vi "NewShooterStateController.vi"(1 "Selected State (In)":string) -> (0 "Selected State (Out)":string)   [LabVIEW 2019]
uses:
  dsinstructions.vi
  outputs.vi
  sensors.vi
  constants.vi
  dsdata.vi
panel:
  in  "Settling Time (ms)":u32=500
  in  "Max Acceptable Robot Speed (ft/s)":dbl=5.0
  in  "Acceptable Shooter Error Fraction":dbl=0.1
  in  "Shooter Prespin (ms)":u32=7000
  in  "Shooter Off Delay (ms)":u32=1000
  in  "Max Range (in)":dbl=1000.0
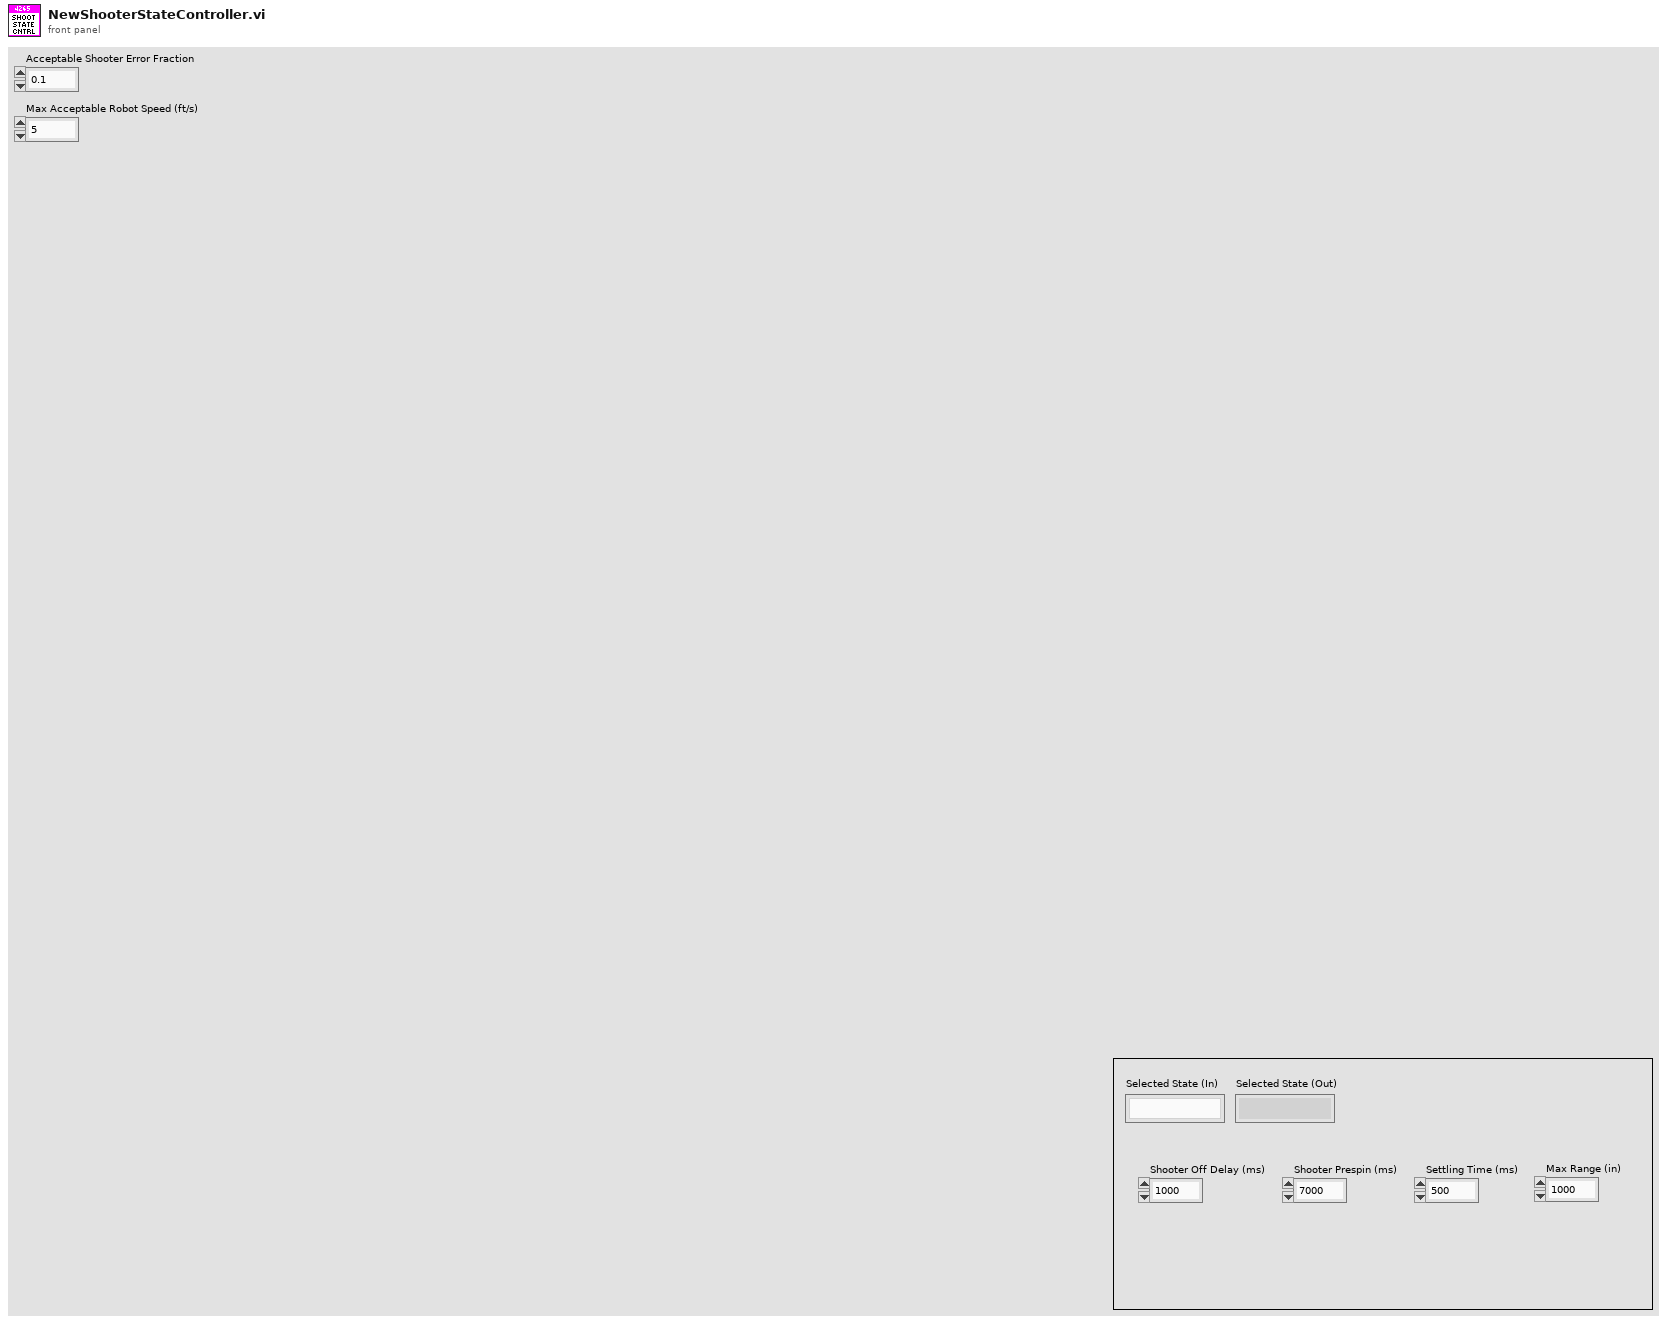
[diagram p1: front panel]
types:
  T1 = enum16{"Center", "North", "NorthWest", "West", "SouthWest", "South", "SouthEast", "East", "NorthEast"}
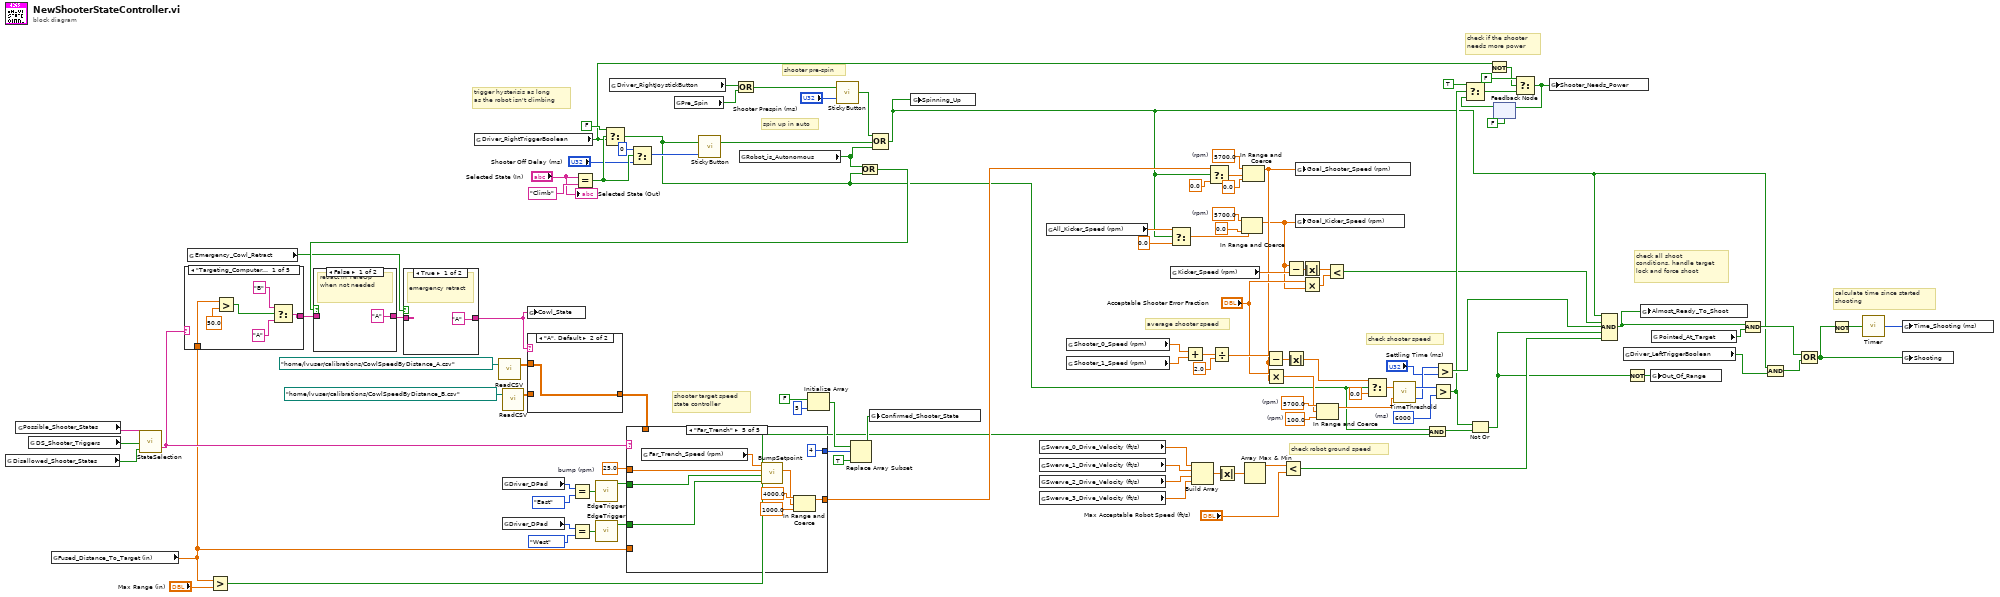
[diagram p0: block diagram]
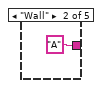
[diagram p4: hidden frame]
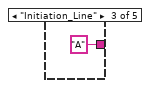
[diagram p5: hidden frame]
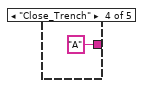
[diagram p6: hidden frame]
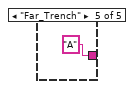
[diagram p7: hidden frame]
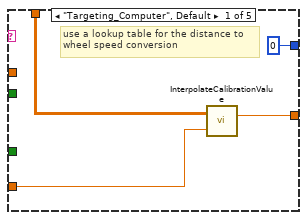
[diagram p9: hidden frame]
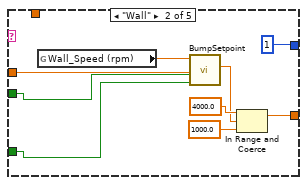
[diagram p10: hidden frame]
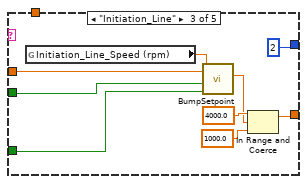
[diagram p11: hidden frame]
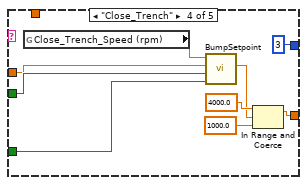
[diagram p12: hidden frame]
diagram:
  w33 = 100.0  # (rpm)
  w34 = 5700.0  # (rpm)
  w42 = 5700.0  # (rpm)
  w5 = 5700.0  # (rpm)
  w45 = u32 6000  # (ms)
  w96 = 25.0  # bump (rpm)
  # "calculate time since started\nshooting"
  # "check all shoot\nconditions, handle target\nlock and force shoot"
  # "average shooter speed"
  # "check shooter speed"
  # "check robot ground speed"
  # "check if the shooter\nneeds more power"
  # "shooter pre-spin"
  # "spin up in auto"
  # "trigger hysterisis as long\nas the robot isn't climbing"
  # "shooter target speed\nstate controller"
  n1 = global read "outputs.vi" "Disallowed_Shooter_States"() -> (w95:bool[])
  n2 = global read "constants.vi" "Possible_Shooter_States"() -> (w113:string[])
  n3 = global read "dsinstructions.vi" "DS_Shooter_Triggers"() -> (w112:bool[])
  n4 = global read "sensors.vi" "Fused_Distance_To_Target (in)"() -> (w86:dbl)
  n5 = call "StateSelection.vi"("Disallowed States"=w95, "State Triggers"=w112, "State Names"=w113) -> ("Selected State"=w87:string)
  n6 = case shown="\"Targeting_Computer\", Default" w87 {
    tunnel: [w114 "A" ("A,B,C") "A" ("A,B,C") "A" ("A,B,C") "A" ("A,B,C")] -> w89
    tunnel: w86 -> [w115 _ _ _ _]
    frame "Targeting_Computer", Default {
      n7 = Greater?(x=w115, y=50.0) -> (0:w119:bool)
      n8 = Select(t="B", s=w119, f="A") -> (s? t:f=w114:string)
    }
    frame "Wall" {
    }
    frame "Initiation_Line" {
    }
    frame "Close_Trench" {
    }
    frame "Far_Trench" {
    }
  }
  n9 = global read "dsdata.vi" "Emergency_Cowl_Retract"() -> (w70:bool)
  n10 = Greater?(x=w86, y="Max Range (in)") -> (0:w20:bool)
  n11 = global read "dsinstructions.vi" "Driver_RightTriggerBoolean"() -> (w63:bool)
  n12 = call "ReadCSV.vi"("File Path (.csv)"=path "/home/lvuser/calibrations/CowlSpeedByDistance_A.csv" ("path")) -> ("Data (index by row)"=w92:dbl[][])  [unwired: 1 in, 1 out]
  n13 = call "ReadCSV.vi"("File Path (.csv)"=path "/home/lvuser/calibrations/CowlSpeedByDistance_B.csv" ("path")) -> ("Data (index by row)"=w91:dbl[][])  [unwired: 1 in, 1 out]
  n14 = global read "dsinstructions.vi" "Driver_DPad"() -> (w104:T1)
  n15 = global read "dsinstructions.vi" "Driver_DPad"() -> (w100:T1)
  n16 = Equal?(x=w104, y=T1."East" ("Driver_DPad")) -> (x = y?=w102:bool)
  n17 = Equal?(x=w100, y=T1."West" ("Driver_DPad")) -> (x = y?=w99:bool)
  n18 = Equal?(x="Selected State (In)", y="Climb") -> (x = y?=w83:bool)
  n19 = call "EdgeTrigger.vi"("Input Signal"=w102) -> ("Rising Edge Trigger"=w101:bool)  [unwired: 2 out]
  n20 = call "EdgeTrigger.vi"("Input Signal"=w99) -> ("Rising Edge Trigger"=w97:bool)  [unwired: 2 out]
  n21 = Select(t=FALSE, s=w83, f=w63) -> (s? t:f=w19:bool)
  n22 = global read "dsinstructions.vi" "Driver_RightJoystickButton"() -> (w78:bool)
  n23 = Select(t=u32 0, s=w83, f="Shooter Off Delay (ms)") -> (s? t:f=w74:u32)
  n24 = global read "dsinstructions.vi" "Pre_Spin"() -> (w79:bool)
  n25 = call "StickyButton.vi"("Time threshold (ms)"=w74, "Button Input"=w19) -> ("Sticky Button"=w73:bool)
  n26 = Or(x=w78, y=w79) -> (x .or. y?=w77:bool)
  n27 = global read "dsdata.vi" "Robot_is_Autonomous"() -> (w72:bool)
  n28 = Initialize Array(FALSE, 5 ("dimension size")) -> (w109:bool[])
  n29 = call "StickyButton.vi"("Time threshold (ms)"="Shooter Prespin (ms)", "Button Input"=w77) -> ("Sticky Button"=w75:bool)
  n30 = Or(x=w72, y=w19) -> (x .or. y?=w71:bool)
  n31 = case shown="False" w71 {
    tunnel: w89 -> [_ w125]
    tunnel: ["A" ("A,B,C") w125] -> w88
    frame False {
      # "retract in TeleOp when not needed"
    }
    frame True {
      # "allow extension in auto and when shooting"
    }
  }
  n32 = case shown="True" w70 {
    tunnel: w88 -> [_ w127]
    tunnel: ["A" ("A,B,C") w127] -> w3
    frame True {
      # "emergency retract"
    }
    frame False {
    }
  }
  n33 = global write "outputs.vi" "Cowl_State"(w3) -> ()
  n34 = case shown="\"A\", Default" w3 {
    tunnel: w92 -> [_ w129]
    tunnel: w91 -> [w128 _]
    tunnel: [w128 w129] -> w90
    frame "B" {
    }
    frame "A", Default {
    }
  }
  n35 = case shown="\"Far_Trench\"" w87 {
    tunnel: [0 1 2 3 4] -> w106
    tunnel: w86 -> [w132 _ _ _ _]
    tunnel: w101 -> [_ w136 w146 w155 w167]
    tunnel: w97 -> [_ w135 w145 w154 w166]
    tunnel: w96 -> [_ w137 w144 w153 w168]
    tunnel: w90 -> [w130 _ _ _ _]
    tunnel: [w131 w134 w143 w152 w161] -> w21
    frame "Targeting_Computer", Default {
      # "use a lookup table for the distance to\nwheel speed conversion"
      n36 = call "InterpolateCalibrationValue.vi"("Input"=w132, "Calibration Data"=w130) -> ("Interpolated Output"=w131:dbl)
    }
    frame "Wall" {
      n37 = global read "dsdata.vi" "Wall_Speed (rpm)"() -> (w141:dbl)
      n38 = call "BumpSetpoint.vi"("Bump Down Trigger"=w135, "Bump Up Trigger"=w136, "Bump Increment"=w137, "Original Setpoint"=w141) -> ("Bumped Setpoint"=w138:dbl)  [unwired: 7 in]
      n39 = In Range and Coerce(upper limit=4000.0, x=w138, lower limit=1000.0) -> (coerced(x)=w134:dbl)  [unwired: 1 out]
    }
    frame "Initiation_Line" {
      n40 = global read "dsdata.vi" "Initiation_Line_Speed (rpm)"() -> (w150:dbl)
      n41 = call "BumpSetpoint.vi"("Bump Down Trigger"=w145, "Bump Up Trigger"=w146, "Bump Increment"=w144, "Original Setpoint"=w150) -> ("Bumped Setpoint"=w147:dbl)  [unwired: 7 in]
      n42 = In Range and Coerce(upper limit=4000.0, x=w147, lower limit=1000.0) -> (coerced(x)=w143:dbl)  [unwired: 1 out]
    }
    frame "Close_Trench" {
      n43 = global read "dsdata.vi" "Close_Trench_Speed (rpm)"() -> (w159:dbl)
      n44 = call "BumpSetpoint.vi"("Bump Down Trigger"=w154, "Bump Up Trigger"=w155, "Bump Increment"=w153, "Original Setpoint"=w159) -> ("Bumped Setpoint"=w156:dbl)  [unwired: 7 in]
      n45 = In Range and Coerce(upper limit=4000.0, x=w156, lower limit=1000.0) -> (coerced(x)=w152:dbl)  [unwired: 1 out]
    }
    frame "Far_Trench" {
      n46 = global read "dsdata.vi" "Far_Trench_Speed (rpm)"() -> (w165:dbl)
      n47 = call "BumpSetpoint.vi"("Bump Down Trigger"=w166, "Bump Up Trigger"=w167, "Bump Increment"=w168, "Original Setpoint"=w165) -> ("Bumped Setpoint"=w162:dbl)  [unwired: 7 in]
      n48 = In Range and Coerce(upper limit=4000.0, x=w162, lower limit=1000.0) -> (coerced(x)=w161:dbl)  [unwired: 1 out]
    }
  }
  n49 = Replace Array Subset(array=w109, new element=TRUE ("new element/subarray"), index=w106) -> (w107:bool[])
  n50 = global write "outputs.vi" "Confirmed_Shooter_State"(w107) -> ()
  n51 = Compound Arithmetic op=OR(w75, w73, w72) -> (w1:bool)
  n52 = global write "outputs.vi" "Spinning_Up"(w1) -> ()
  n53 = global read "sensors.vi" "Swerve_0_Drive_Velocity (ft/s)"() -> (w54:dbl)
  n54 = global read "sensors.vi" "Swerve_1_Drive_Velocity (ft/s)"() -> (w53:dbl)
  n55 = global read "sensors.vi" "Swerve_2_Drive_Velocity (ft/s)"() -> (w52:dbl)
  n56 = global read "sensors.vi" "Swerve_3_Drive_Velocity (ft/s)"() -> (w51:dbl)
  n57 = global read "dsdata.vi" "All_Kicker_Speed (rpm)"() -> (w40:dbl)
  n58 = global read "sensors.vi" "Shooter_0_Speed (rpm)"() -> (w60:dbl)
  n59 = global read "sensors.vi" "Shooter_1_Speed (rpm)"() -> (w59:dbl)
  n60 = Select(t=w40, s=w1, f=0.0) -> (s? t:f=w39:dbl)
  n61 = global read "sensors.vi" "Kicker_Speed (rpm)"() -> (w38:dbl)
  n62 = Add(x=w60, y=w59) -> (x+y=w58:dbl)
  n63 = Build Array(w54, w53, w52, w51) -> (w50:dbl[])
  n64 = Select(t=w21, s=w1, f=0.0) -> (s? t:f=w44:dbl)
  n65 = Divide(x=w58, y=2.0) -> (x/y=w55:dbl)
  n66 = Absolute Value(x=w50) -> (abs(x)=w49:dbl[])
  n67 = In Range and Coerce(upper limit=w42, x=w39, lower limit=0.0) -> (coerced(x)=w22:dbl)  [unwired: 1 out]
  n68 = In Range and Coerce(upper limit=w5, x=w44, lower limit=0.0) -> (coerced(x)=w29:dbl)  [unwired: 1 out]
  n69 = Array Max & Min(array=w49) -> (max value=w48:dbl)  [unwired: 3 out]
  n70 = Subtract(x=w55, y=w29) -> (x-y=w56:dbl)
  n71 = Multiply(x="Acceptable Shooter Error Fraction", y=w29) -> (x*y=w32:dbl)
  n72 = Less?(x=w48, y="Max Acceptable Robot Speed (ft/s)") -> (x < y?=w8:bool)
  n73 = Subtract(x=w22, y=w38) -> (x-y=w37:dbl)
  n74 = Absolute Value(x=w56) -> (abs(x)=w28:dbl)
  n75 = global write "outputs.vi" "Goal_Shooter_Speed (rpm)"(w29) -> ()
  n76 = global write "outputs.vi" "Goal_Kicker_Speed (rpm)"(w22) -> ()
  n77 = Absolute Value(x=w37) -> (abs(x)=w30:dbl)
  n78 = Multiply(x="Acceptable Shooter Error Fraction", y=w22) -> (x*y=w35:dbl)
  n79 = In Range and Coerce(upper limit=w34, x=w32, lower limit=w33) -> (coerced(x)=w31:dbl)  [unwired: 1 out]
  n80 = Less?(x=w30, y=w35) -> (x < y?=w2:bool)
  n81 = Select(t=w28, s=w19, f=0.0) -> (s? t:f=w27:dbl)
  n82 = call "TimeThreshold.vi"("Threshold"=w31, "Current Value"=w27) -> ("Time Below Threshold (ms)"=w24:u32, "Time Above Threshold (ms)"=w46:u32)
  n83 = And(x=w19, y=w20) -> (x .and. y?=w25:bool)
  n84 = Greater?(x=w46, y=w45) -> (0:w6:bool)
  n85 = Greater?(x=w24, y="Settling Time (ms)") -> (0:w9:bool)
  n86 = Not Or(1:w25, 2:w6) -> (0:w4:bool)
  n87 = Not(x=w63) -> (.not. x?=w64:bool)
  n88 = feedback #1(FALSE) -> (w68:bool)
  n89 = Select(t=TRUE, s=w6, f=w68) -> (s? t:f=w67:bool)
  n90 = Select(t=FALSE, s=w64, f=w67) -> (s? t:f=w65:bool)
  n91 = feedback-in #1(w65) -> ()
  n92 = global write "outputs.vi" "Shooter_Needs_Power"(w65) -> ()
  n93 = Compound Arithmetic op=AND(w1, w2, w9, w4, w8) -> (w15:bool)
  n94 = global read "dsinstructions.vi" "Driver_LeftTriggerBoolean"() -> (w14:bool)
  n95 = Not(x=w4) -> (.not. x?=w16:bool)
  n96 = global write "outputs.vi" "Almost_Ready_To_Shoot"(w15) -> ()
  n97 = global write "outputs.vi" "Out_Of_Range"(w16) -> ()
  n98 = global read "sensors.vi" "Pointed_At_Target"() -> (w17:bool)
  n99 = Compound Arithmetic op=AND(w15, w17) -> (w18:bool)
  n100 = Compound Arithmetic op=AND(w1, w14) -> (w13:bool)
  n101 = Compound Arithmetic op=OR(w18, w13) -> (w12:bool)
  n102 = Not(x=w12) -> (.not. x?=w11:bool)
  n103 = call "Timer.vi"("Reset Timer"=w11) -> ("Time (ms)"=w10:u32)
  n104 = global write "outputs.vi" "Time_Shooting (ms)"(w10) -> ()
  n105 = global write "outputs.vi" "Shooting"(w12) -> ()
  "Selected State (Out)" <- "Selected State (In)"
